vi "Insert Namespace.vi"(4 "Test File Version Number":string, 8 "error in (no error)":errorcluster, 9 "Linked List ID":string, 10 "Name":string, 11 "Custom Type Test Executive in":refnum<class "Custom Type Test Executive.lvclass">) -> (0 "error out":errorcluster, 1 "Replaced?":bool, 3 "Custom Type Test Executive out":refnum<class "Custom Type Test Executive.lvclass">, 5 "Unique ID out":string)   [LabVIEW 2017, in "Custom Type Test Executive.lvlib" / "Custom Type Test Executive.lvclass"]
uses:
  <vilib>/gpm_packages/@cs/test-executive/Source/Custom Type Test Executive/Custom Type Test Executive/Custom Type Test Executive.lvclass
  C:/Program Files/National Instruments/LabVIEW 2017/vi.lib/gpm_packages/@cs/test-executive/Source/Test Executive/TestExecutive/Test Executive.lvclass
  <vilib>/gpm_packages/@cs/test-executive/Source/Test Executive/Name Space/Name Space.lvclass
  <vilib>/gpm_packages/@cs/data-type-serializer/source/Boolean/Boolean.lvclass/Boolean.ctl
  <vilib>/gpm_packages/@cs/test-executive/Source/Test Executive/TestExecutive/Test Executive.lvclass/Test Executive.ctl
  449b78f0-b227-40dc-a1b5-3a86b1d7352f.vi
  <vilib>/gpm_packages/@cs/data-type-serializer/source/Boolean/Boolean.lvclass
  <vilib>/gpm_packages/@cs/linked-list/Source/Linked List/ILinkedList/ILinked List.lvclass
  <vilib>/gpm_packages/@cs/linked-list/Source/Linked List/Linked List Ref/Linked List Ref.lvclass
  <vilib>/gpm_packages/@cs/test-executive/Source/Test Executive/TestExecutive/Test Executive.lvclass
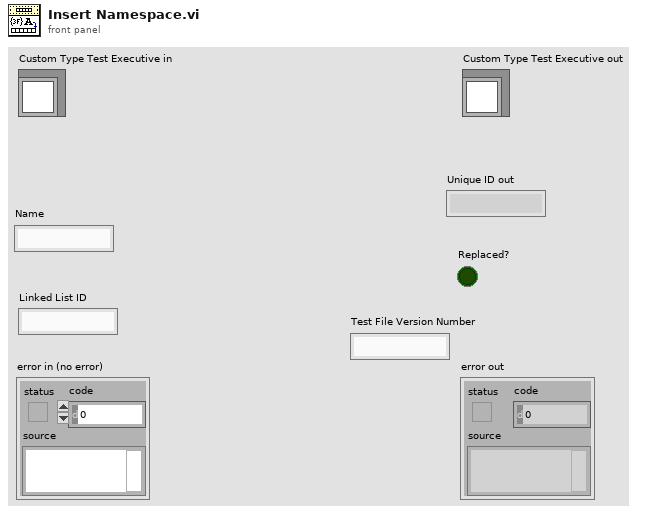
[diagram p1: front panel]
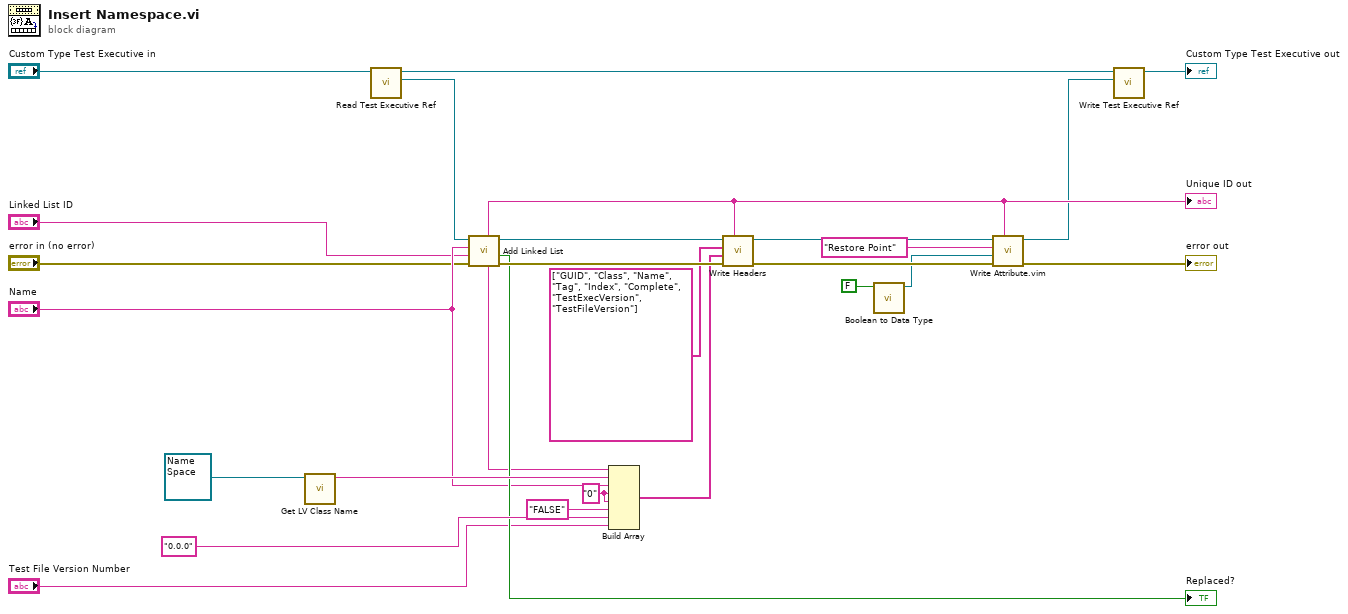
[diagram p0: block diagram]
diagram:
  w19 = "0" ("element")
  n1 = call <vilib>:"Get LV Class Name.vi"("object"=refnum<class "Name Space.lvclass"> refnum ("Test Executive.lvlib:Name Space.lvclass")) -> ("class name"=w21:string)  [unwired: 9 in, 1 out]
  n2 = call <vilib>:"Read Test Executive Ref.vi"("Test Executive in"="Custom Type Test Executive in") -> ("Test Executive Ref"=w7:refnum<data-value>, "Test Executive out"=w8:refnum<class "Custom Type Test Executive.lvclass">)  [unwired: 9 in]
  n3 = call <vilib>:"Add Linked List.vi"("error in (no error)"="error in (no error)", "Linked List ID"="Linked List ID", "Name"="Name", "Linked List Ref"=w7) -> ("error out"=w25:errorcluster, "Replaced?"=→"Replaced?":bool, "Linked List Ref out"=w26:refnum<data-value>, "Linked List ID out"=w12:string)  [unwired: 4 in]
  "Unique ID out" <- w12
  n4 = Build Array(w12, w21, "Name", w19, w19, "FALSE" ("element"), "0.0.0" ("Test Executive Version Number"), "Test File Version Number") -> (w23:string[])
  n5 = call <vilib>:"Write Headers.vi"("Linked List ID"=w12, "error in (no error)"=w25, "Header Values"=w23, "Header Names"=string[] ["GUID", "Class", "Name", "Tag", "Index", "Complete", "TestExecVersion", "TestFileVersion"], "Linked List Ref"=w26) -> ("error out"=w16:errorcluster, "Linked List Ref out"=w17:refnum<data-value>)  [unwired: 5 in]
  n6 = call <vilib>:"Boolean to Data Type.vi"("Boolean"=FALSE) -> ("Boolean out"=w1:refnum<class "Boolean.lvclass">)  [unwired: 9 in, 1 out]
  n7 = call "Write Attribute.vim"("Linked List ID"=w12, "error in (no error)"=w16, "Attribute"=w1, "Attribute Name"="Restore Point", "Linked List Ref"=w17) -> ("error out"=→"error out":errorcluster, "Linked List Ref out"=w10:refnum<data-value>)  [unwired: 3 in, 2 out]
  n8 = call <vilib>:"Write Test Executive Ref.vi"("Test Executive Ref"=w10, "Test Executive in"=w8) -> ("Test Executive out"=→"Custom Type Test Executive out":refnum<class "Custom Type Test Executive.lvclass">)  [unwired: 9 in]
